vi "onHttpPost (Multipart).vi"(6 "timeout":i32=10000, 7 "output file":path, 8 "error in":errorcluster, 9 "Multipart Post data":T1[](array[typedef]), 10 "url":string, 11 "advanced-http-client in":refnum<class "advanced-http-client.lvclass">) -> (0 "error out":errorcluster, 1 "body":string, 2 "headers":string, 3 "advanced-http-client out":refnum<class "advanced-http-client.lvclass">)   [LabVIEW 2020, in "advanced-http-client.lvclass"]
uses:
  advanced-http-client.lvclass
  <vilib>/httpClient/MultipartData.ctl
  advanced-http-client.lvclass/advanced-http-client.ctl
  <vilib>/NI/Advanced HTTP Client/POST (Multipart).vi
  <vilib>/NI/Advanced HTTP Client/Session.lvclass
  <vilib>/httpClient/LabVIEWHTTPClient.lvlib
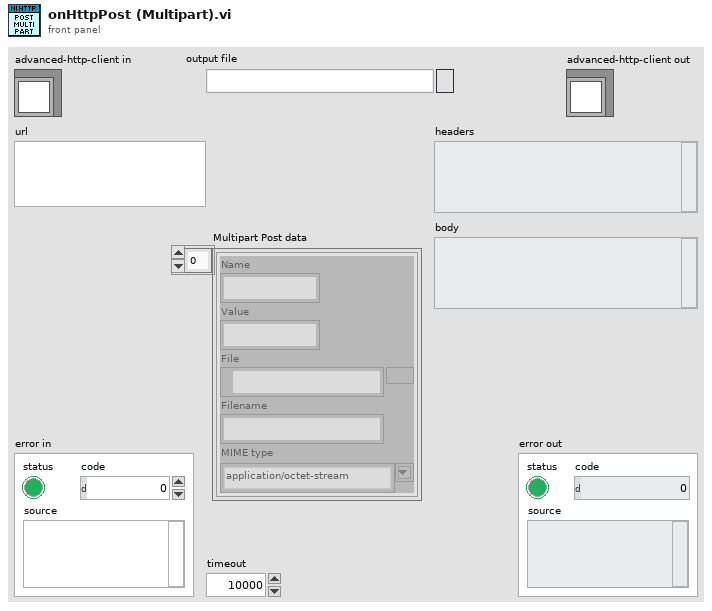
[diagram p1: front panel]
types:
  T1 = typedef "LabVIEWHTTPClient.lvlib/MultipartData.ctl" = cluster{"Name":string, "Value":string, "File":path, "Filename":string, "MIME type":string}
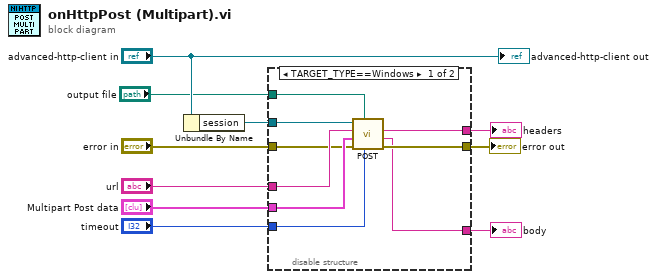
[diagram p0: block diagram]
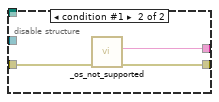
[diagram p2: hidden frame]
diagram:
  n1 = Unbundle By Name("advanced-http-client in") -> ("session"=w9:refnum<class "Session.lvclass">)
  n2 = disable-structure shown="TARGET_TYPE==Windows" {
    disable-tunnel: w9 -> [w19 _]
    disable-tunnel: "url" -> [w18 _]
    disable-tunnel: "Multipart Post data" -> [w17 _]
    disable-tunnel: "error in" -> [w16 w22]
    disable-tunnel: [w15 w21] -> w5
    disable-tunnel: [w14 w20] -> w4
    disable-tunnel: [w13 _] -> w3
    disable-tunnel: "timeout" -> [w12 _]
    disable-tunnel: "output file" -> [w11 _]
    frame condition #0 (active) {
      n3 = call-poly <vilib>:"POST.vi"("timeout"=w12, "output file"=w11, "error in"=w16, "data"=w17, "url"=w18, "session in"=w19) -> ("error out"=w15:errorcluster, "body"=w13:string, "headers"=w14:string)  [unwired: 1 in, 2 out]
    }
    frame condition #1 {
      n4 = call "_os_not_supported.vi"("error in (no error)"=w22) -> ("error out"=w21:errorcluster, "headers"=w20:string)  [unwired: 9 in]
    }
  }
  "error out" <- w5
  "headers" <- w4
  "body" <- w3
  "advanced-http-client out" <- "advanced-http-client in"
